vi "Call_MATLAB_Suite.vi"(0 "Mode":T1, 1 "Input String":string) -> (3 "MatLab Finished Character?":bool, 4 "Output file":path, 5 "error out":errorcluster)   [LabVIEW 2021]
uses:
  MATLAB_Mode.ctl
  Anemometry/Anemometry Sub Vis/Globals/Constants_global.vi
panel:
  out "return code":i32
  out "auditTrail":string[](array[string])
  out "steps":i32
  out "startup command":string
  out "startup standard error":string
  out "startup standard output":string
  out "Seconds":dbl
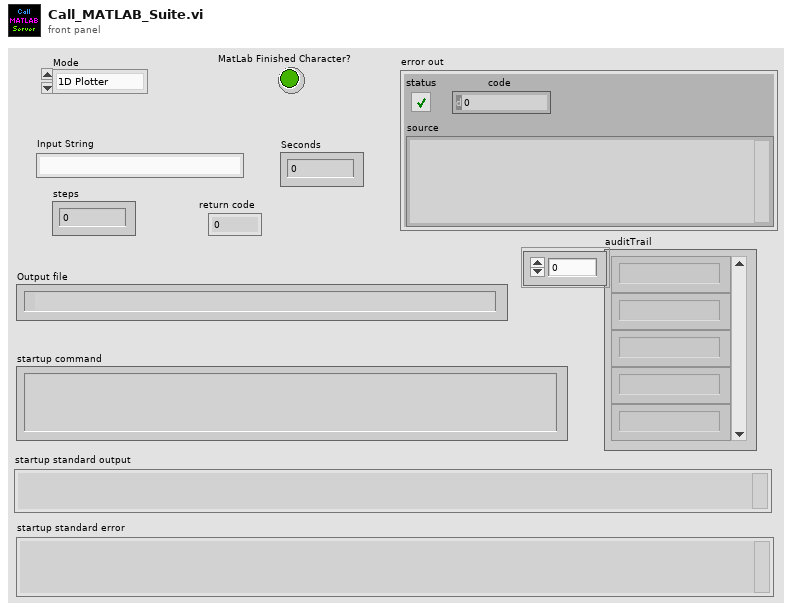
[diagram p1: front panel]
types:
  T1 = typedef "MATLAB_Mode.ctl" = enum16{"1D Plotter", "2D Plotter", "LP Plotter", "7HP UVW"}
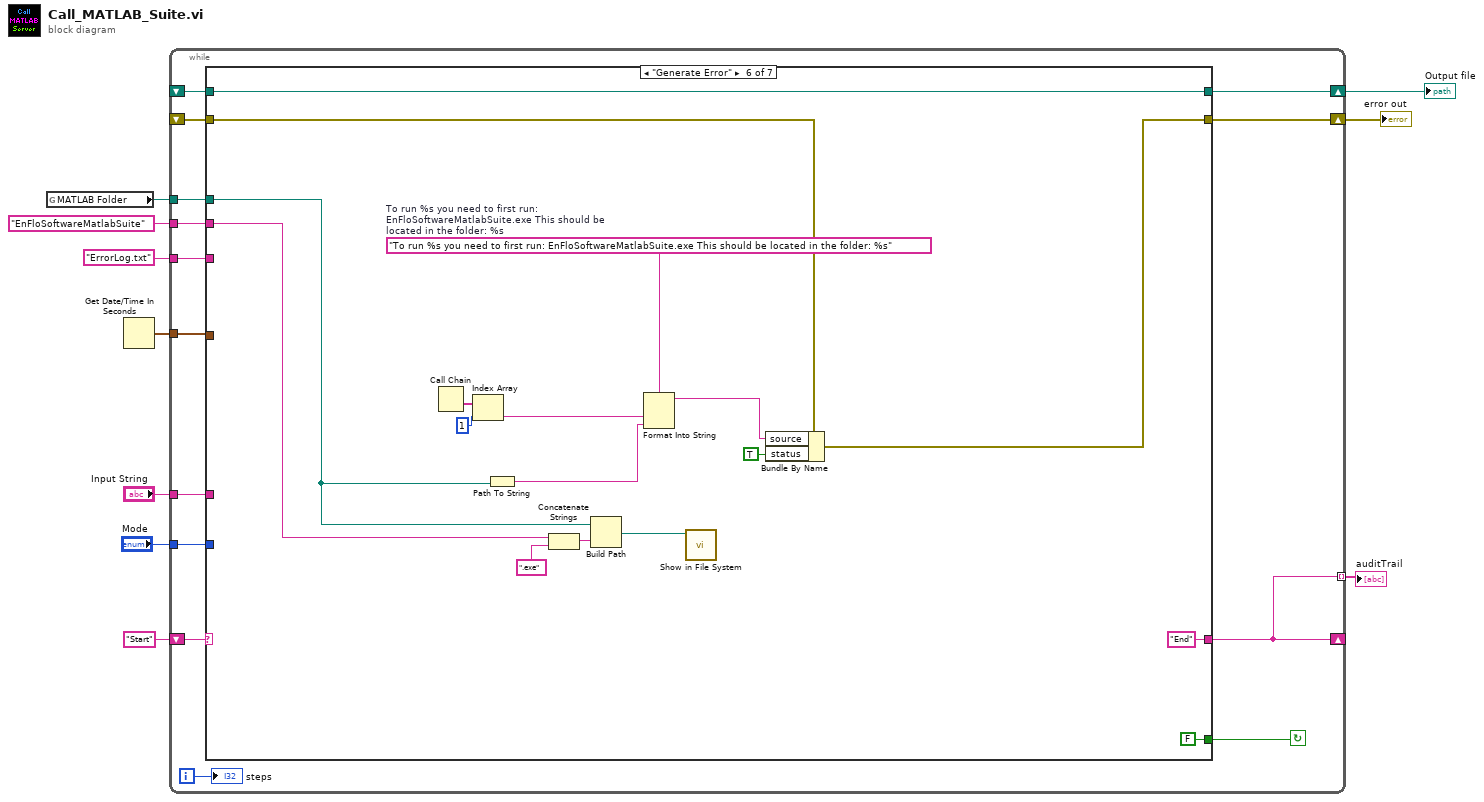
[diagram p0: block diagram]
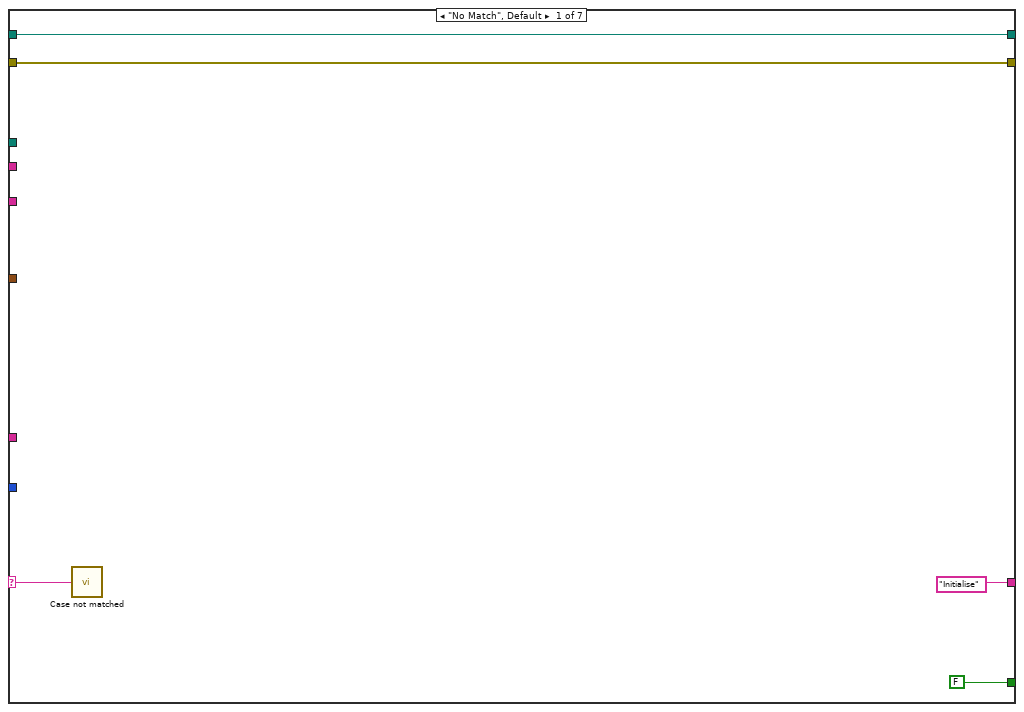
[diagram p2: hidden frame]
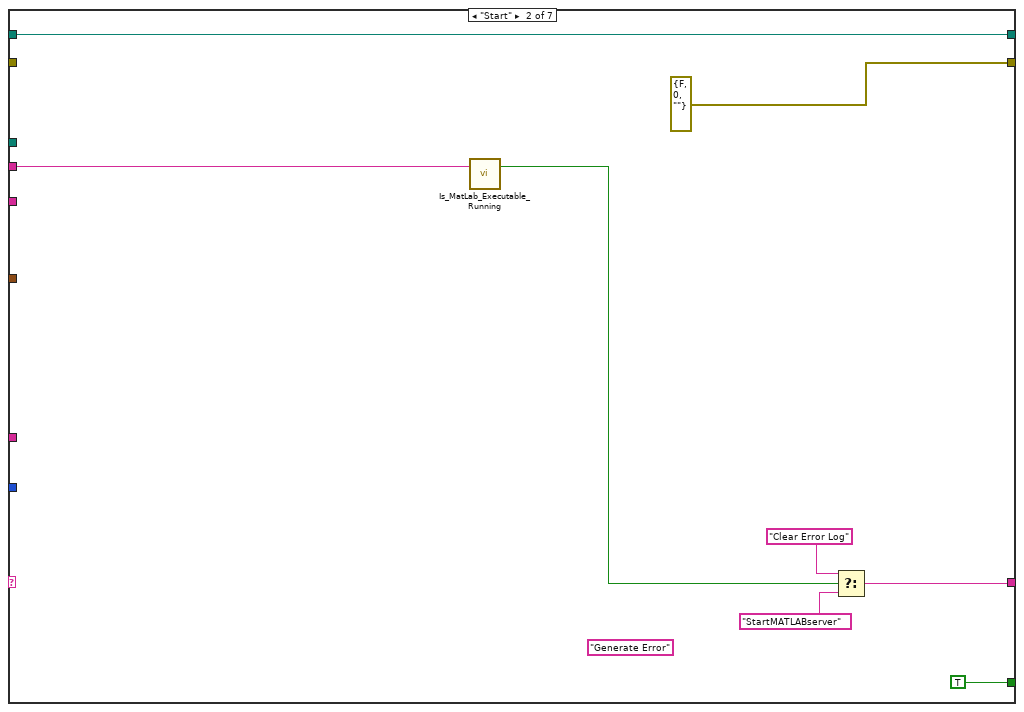
[diagram p3: hidden frame]
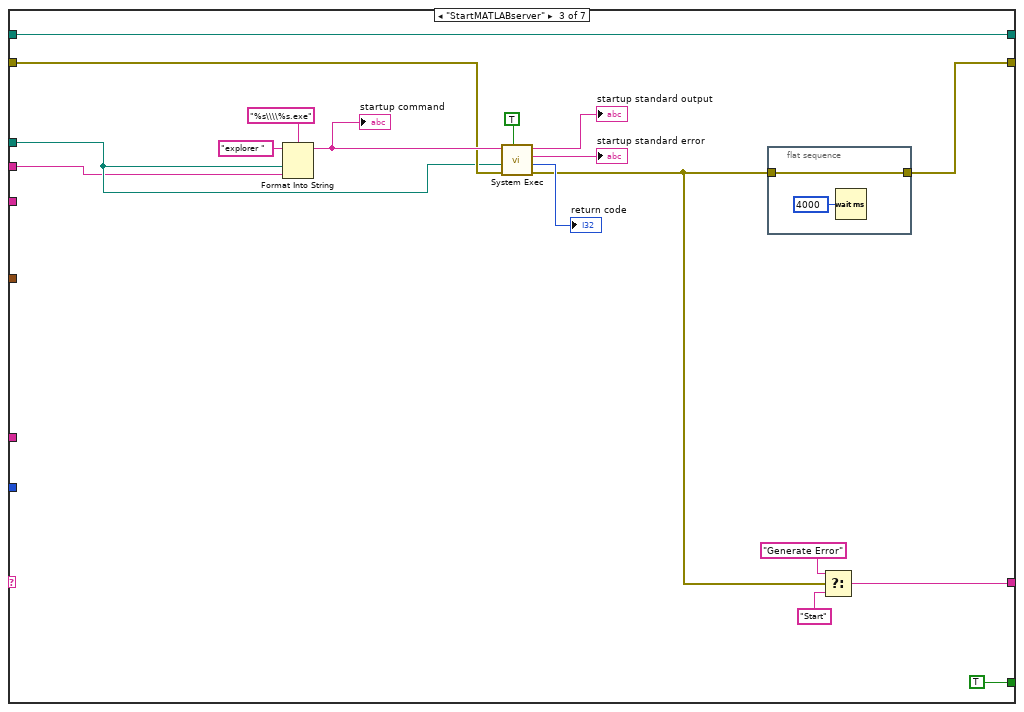
[diagram p4: hidden frame]
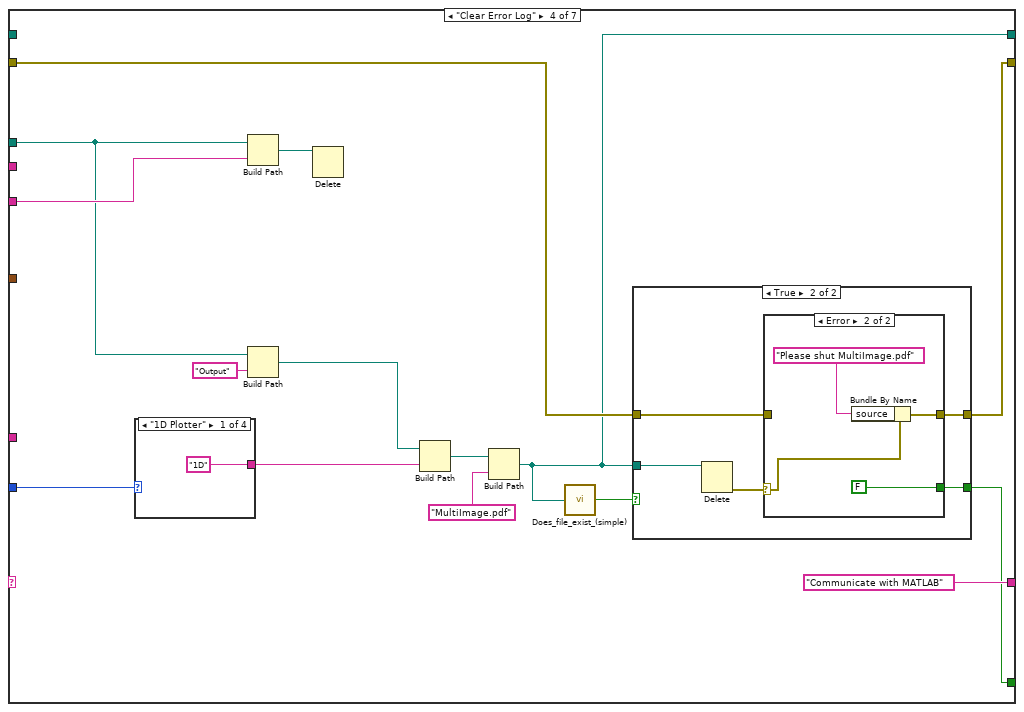
[diagram p5: hidden frame]
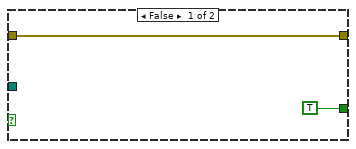
[diagram p6: hidden frame]
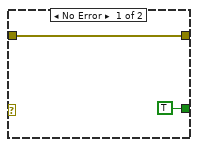
[diagram p7: hidden frame]
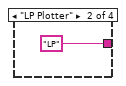
[diagram p8: hidden frame]
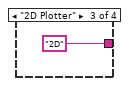
[diagram p9: hidden frame]
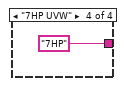
[diagram p10: hidden frame]
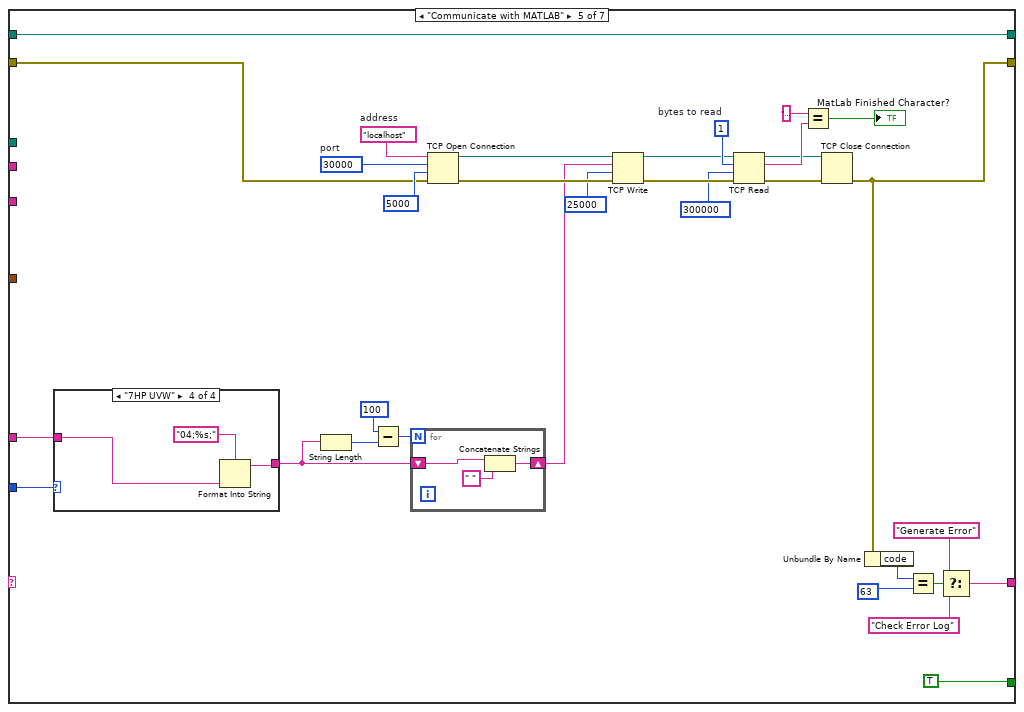
[diagram p11: hidden frame]
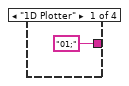
[diagram p12: hidden frame]
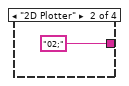
[diagram p13: hidden frame]
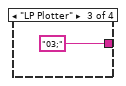
[diagram p14: hidden frame]
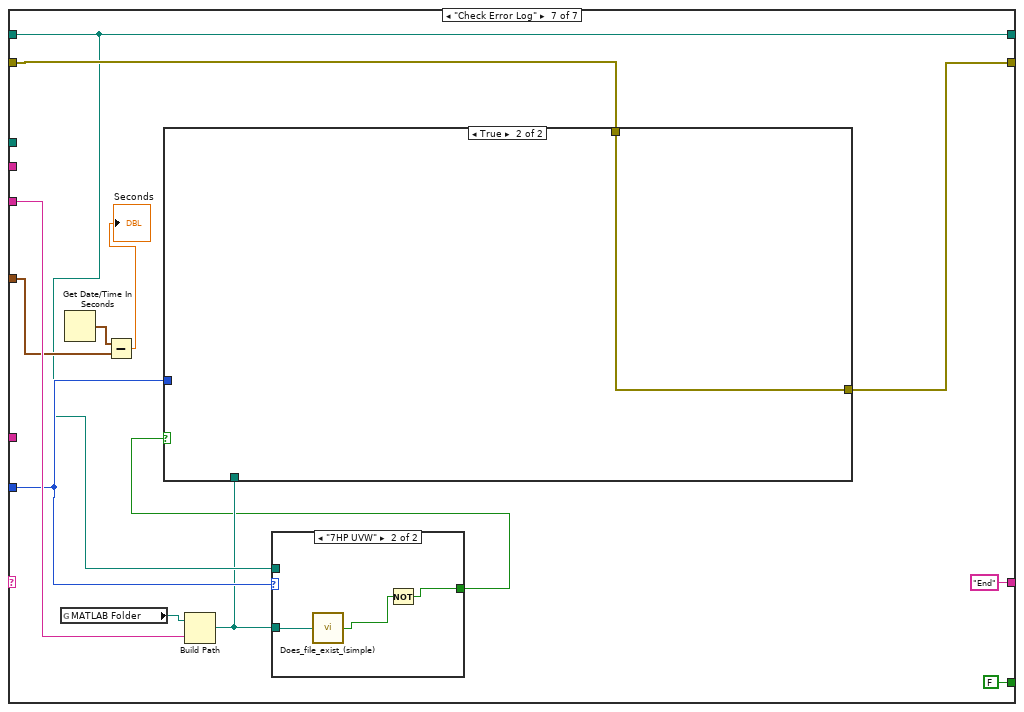
[diagram p15: hidden frame]
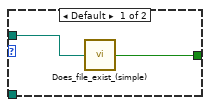
[diagram p16: hidden frame]
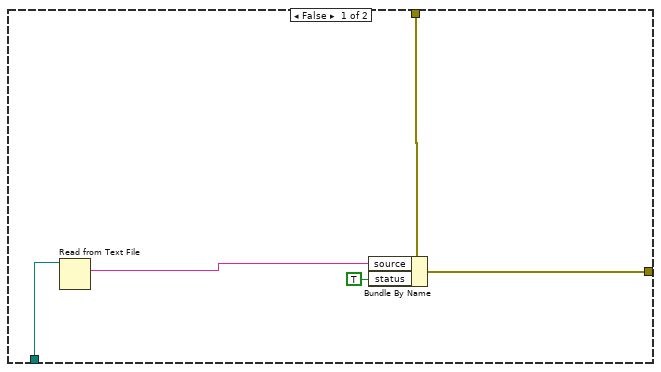
[diagram p17: hidden frame]
diagram:
  n1 = global read "Constants_global.vi" "MATLAB Folder"() -> (w6:path)
  n2 = Get Date/Time In Seconds() -> (seconds since 1Jan1904=w5:timestamp)
  n3 = while {
    shift-left: "Start" -> [w24]
    shift-right: [w11] -> _
    tunnel: "ErrorLog.txt" ("name or relative path") -> [w23]
    shift-right: [w14] -> w3
    shift-left: _ -> [w22]
    tunnel: "Mode" -> [w20]
    tunnel: "Input String" -> [w19]
    shift-right: [w18] -> w4
    shift-left: _ -> [w17]
    tunnel: w6 -> [w16]
    tunnel: w5 -> [w15]
    tunnel: "EnFloSoftwareMatlabSuite" ("executable") -> [w13]
    tunnel: [w11] -> w1 mode=indexing
    i -> [w12]
    stop <- w21 continue-if-true
    n4 = case shown="\"Generate Error\"" w24 {
      selector: w24 -> [w25 _ _ _ _ _ _]
      tunnel: [FALSE TRUE TRUE w61 TRUE FALSE FALSE] -> w21
      tunnel: ["Initialise" w34 w40 "Communicate with MATLAB" w90 "End" ("f") "End" ("f")] -> w11
      tunnel: w23 -> [_ _ _ w69 _ _ w154]
      tunnel: [w27 errorcluster {"status"=FALSE, "code"=0, "source"=""} ("error in (no error)") w47 w60 w94 w142 w159] -> w14
      tunnel: w22 -> [w27 _ w52 w59 w96 w141 w158]
      tunnel: w20 -> [_ _ _ w68 w107 _ w150]
      tunnel: w19 -> [_ _ _ _ w101 _ _]
      tunnel: [w26 w32 w54 w58 w100 w135 w149] -> w18
      tunnel: w17 -> [w26 w32 w54 _ w100 w135 w149]
      tunnel: w16 -> [_ _ w44 w57 _ w133 _]
      tunnel: w15 -> [_ _ _ _ _ _ w152]
      tunnel: w13 -> [_ w31 w43 _ _ w130 _]
      frame "No Match", Default {
        n5 = call "Case not matched.vi"("Case Name not Matched"=w25) -> ()
      }
      frame "Start" {
        (unwired) "Generate Error" ("f")
        n6 = call "Is_MatLab_Executable_Running.vi"("executable"=w31) -> ("Running?"=w36:bool)  [unwired: 1 in, 1 out]
        n7 = Select(t="Clear Error Log", s=w36, f="StartMATLABserver") -> (s? t:f=w34:string)
      }
      frame "StartMATLABserver" {
        n8 = Format Into String(format string="%s\\\\%s.exe", initial string="explorer ", w44, w43) -> (resulting string=w53:string)  [unwired: 1 in, 1 out]
        "startup command" <- w53
        n9 = call <vilib>:"System Exec.vi"("wait until completion? (T)"=TRUE, "error in (no error)"=w52, "working directory"=w44, "command line"=w53) -> ("error out"=w42:errorcluster, "return code"=→"return code":i32, "standard error"=→"startup standard error":string, "standard output"=→"startup standard output":string)  [unwired: 4 in]
        n10 = flat-sequence {
          tunnel: w42 -> [w55]
          tunnel: [w55] -> w47
          frame #0 {
            n11 = Wait (ms)(milliseconds to wait=u32 4000) -> ()  [unwired: 1 out]
          }
        }
        n12 = Select(t="Generate Error", s=w42, f="Start") -> (s? t:f=w40:string)
      }
      frame "Clear Error Log" {
        n13 = case shown="\"1D Plotter\"" w68 {
          tunnel: ["1D" "LP" "2D" "7HP"] -> w65
          frame "1D Plotter" {
          }
          frame "LP Plotter" {
          }
          frame "2D Plotter" {
          }
          frame "7HP UVW" {
          }
        }
        n14 = Build Path(base path=w57, name or relative path=w69) -> (appended path=w70:path)
        n15 = Build Path(base path=w57, name or relative path="Output") -> (appended path=w66:path)
        n16 = Delete(path (use dialog)=w70) -> ()  [unwired: 4 in, 3 out]
        n17 = Build Path(base path=w66, name or relative path=w65) -> (appended path=w64:path)
        n18 = Build Path(base path=w64, name or relative path="MultiImage.pdf") -> (appended path=w58:path)
        n19 = call "Does_file_exist_(simple).vi"("Pathname"=w58) -> ("exists?"=w62:bool)
        n20 = case shown="True" w62 {
          tunnel: w58 -> [_ w78]
          tunnel: [TRUE w76] -> w61
          tunnel: [w72 w75] -> w60
          tunnel: w59 -> [w72 w74]
          frame False {
          }
          frame True {
            n21 = Delete(path (use dialog)=w78) -> (error out=w77:errorcluster)  [unwired: 4 in, 2 out]
            n22 = case shown="Error" w77 {
              selector: w77 -> [_ w83]
              tunnel: [TRUE FALSE] -> w76
              tunnel: [w79 w82] -> w75
              tunnel: w74 -> [w79 _]
              frame No Error {
              }
              frame Error {
                n23 = Bundle By Name(cluster=w83, "source"="Please shut MultiImage.pdf" ("message")) -> (w82:errorcluster)
              }
            }
          }
        }
      }
      frame "Communicate with MATLAB" {
        w99 = u16 30000  # port
        w98 = "localhost"  # address
        w110 = 1  # bytes to read
        n24 = case shown="\"7HP UVW\"" w107 {
          tunnel: ["01;" ("format string") "02;" ("format string") "03;" ("format string") w127] -> w103
          tunnel: w101 -> [_ _ _ w128]
          frame "1D Plotter" {
          }
          frame "2D Plotter" {
          }
          frame "LP Plotter" {
          }
          frame "7HP UVW" {
            n25 = Format Into String(format string="04;%s;", w128) -> (resulting string=w127:string)  [unwired: 2 in, 1 out]
          }
        }
        n26 = String Length(string=w103) -> (length=w105:i32)
        n27 = Subtract(x=100, y=w105) -> (x-y=w106:i32)
        n28 = for {
          N: w106 -> [_]
          shift-right: [w123] -> w102
          shift-left: w103 -> [w121]
          n29 = Concatenate Strings(w121, " ") -> (w123:string)
        }
        n30 = TCP Open Connection(address=w98, remote port or service name=w99, timeout ms (60000)=5000, error in (no error)=w96) -> (connection ID=w112:refnum<k5>, error out=w119:errorcluster)  [unwired: 1 in]
        n31 = TCP Write(connection ID=w112, data in=w102, error in (no error)=w119, 9:25000 ("timeout ms (25000)")) -> (connection ID out=w109:refnum<k5>, error out=w114:errorcluster)  [unwired: 1 out]
        n32 = TCP Read(connection ID=w109, bytes to read=w110, error in (no error)=w114, 9:300000 ("timeout ms (25000)")) -> (connection ID out=w115:refnum<k5>, data out=w117:string, error out=w113:errorcluster)  [unwired: 1 out]
        n33 = Equal?(x="\u0001" ("Reply from Matlab"), y=w117) -> (x = y?=→"MatLab Finished Character?":bool)
        n34 = TCP Close Connection(connection ID=w115, error in (no error)=w113) -> (error out=w94:errorcluster)  [unwired: 1 in, 1 out]
        n35 = Unbundle By Name(w94) -> ("code"=w93:i32)
        n36 = Equal?(x=w93, y=63) -> (x = y?=w92:bool)
        n37 = Select(t="Generate Error", s=w92, f="Check Error Log") -> (s? t:f=w90:string)
      }
      frame "Generate Error" {
        w145 = "To run %s you need to first run: EnFloSoftwareMatlabSuite.exe This should be located in the folder: %s"  # To run %s you need to first run: EnFloSoftwareMatlabSuite.exe This should be located in the folder: %s
        n38 = Call Chain() -> (call chain=w137:string[])
        n39 = Index Array(array=w137, index=1 ("Index")) -> (element=w136:string)
        n40 = Path To String(path=w133) -> (string=w143:string)
        n41 = Concatenate Strings(w130, ".exe") -> (w132:string)
        n42 = Build Path(base path=w133, name or relative path=w132) -> (appended path=w134:path)
        n43 = Format Into String(format string=w145, w136, w143) -> (resulting string=w146:string)  [unwired: 2 in, 1 out]
        n44 = call <vilib>:"Show in File System.vi"("file or directory path"=w134) -> ()  [unwired: 10 in, 1 out]
        n45 = Bundle By Name(cluster=w141, "source"=w146, "status"=TRUE) -> (w142:errorcluster)
      }
      frame "Check Error Log" {
        n46 = global read "Constants_global.vi" "MATLAB Folder"() -> (w155:path)
        n47 = Get Date/Time In Seconds() -> (seconds since 1Jan1904=w153:timestamp)
        n48 = Subtract(x=w153, y=w152) -> (x-y=→"Seconds":dbl)
        n49 = Build Path(base path=w155, name or relative path=w154) -> (appended path=w148:path)
        n50 = case shown="\"7HP UVW\"" w150 {
          tunnel: w149 -> [w161 _]
          tunnel: w148 -> [_ w164]
          tunnel: [w160 w162] -> w147
          frame Default {
            n51 = call "Does_file_exist_(simple).vi"("Pathname"=w161) -> ("exists?"=w160:bool)
          }
          frame "7HP UVW" {
            n52 = call "Does_file_exist_(simple).vi"("Pathname"=w164) -> ("exists?"=w163:bool)
            n53 = Not(x=w163) -> (.not. x?=w162:bool)
          }
        }
        n54 = case shown="True" w147 {
          tunnel: [w168 w170] -> w159
          tunnel: w158 -> [w167 w170]
          tunnel: w148 -> [w166 _]
          tunnel: w150 -> [_ _]
          frame False {
            n55 = Read from Text File(file (use dialog)=w166) -> (text=w165:string)  [unwired: 3 in, 3 out]
            n56 = Bundle By Name(cluster=w167, "source"=w165, "status"=TRUE) -> (w168:errorcluster)
          }
          frame True {
          }
        }
      }
    }
    "steps" <- w12
  }
  "error out" <- w3
  "Output file" <- w4
  "auditTrail" <- w1
